vi "Stoerung Durchfluss FT-IR.vi"(10 "Durchfluss FT-IR":sgl) -> (0 "AbschMax":bool, 1 "AbschMin":bool, 2 "WarnMax":bool, 3 "WarnMin":bool, 5 "F.Br.":bool)   [LabVIEW 2020, in "Stoermeldungen.lvlib"]
uses:
  Stoermeldungen.lvlib
  Allgemein/FGV Analysator aktiv.ctl
  Aktion Anlagengrenzen pruefen.ctl
  Allgemein/FGV Zustaende Aktionen.ctl
  Seiten/Anlagengrenzwerte/Anlagen-Parameternamen.ctl
  Allgemein/Allgemein.lvlib
  Seiten/Anlagengrenzwerte/Anlagengrenzwerte.lvlib
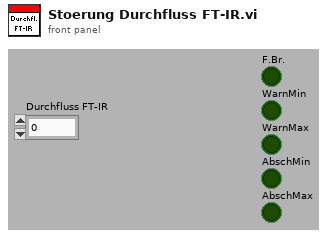
[diagram p1: front panel]
types:
  T1 = typedef "Allgemein.lvlib/FGV Analysator aktiv.ctl" = enum16{"lesen", "Analysator", "CG Aufschaltung", "KAL Zustand", "AutaKal GT?"}
  T2 = typedef "CalGas Aufschaltung.lvlib/Aufschaltung CalGas.ctl" = cluster{"Kalibriergas":T3, "Aufschaltpunkt":T4, "Analysator":T5}
  T3 = typedef "Auswahlfeld.ctl" = u16
  T4 = typedef "CalGas Aufschaltung.lvlib/Auswahl Aufschaltpunkt.ctl" = enum16{"über Filterblock", "Analysator direkt", "über PNS", "Entnahme", "Gasdivider"}
  T5 = typedef "CalGas Aufschaltung.lvlib/Auswahl Analysator.ctl" = enum16{"FT-IR", "FID", "PMA", "PMA/FID/FT-IR"}
  T6 = typedef "Status Analysatoren.lvlib/Status Analysatoren_Anzeige.ctl" = cluster{"FT-IR":bool, "FID":bool, "PMA":bool}
  T7 = typedef "Anlagengrenzwerte.lvlib/Anlagen-Parameternamen.ctl" = enum16{"Eingangsdruck FT-IR:", "Durchfluss FT-IR:", "Durchfluss CalGas", "Druck Ausgang", "Druck Kalter Block", "Heizleitung intern", "Heizleitung zu FT-IR", "Heizung Filter:", "Heizung Pumpe:", "HL Extern SP1", "HL Extern SP2", "FT-IR Messzelle", "Schaltschrank", "Gaskühler"}
  T8 = typedef "Allgemein.lvlib/FGV Zustaende Aktionen.ctl" = enum16{"lesen", "Zustand PC", "Zustand cRIO", "Bildnummer", "Samplepoint", "Sysloglevel"}
  T9 = typedef "Stoermeldungen.lvlib/Aktion Anlagengrenzen pruefen.ctl" = enum16{"Temp.", "HKL", "Druck", "SS Temp."}
  T10 = typedef "Funktionstasten.lvlib/Zustaende.ctl" = enum16{"Standby", "Pause", "Eco", "Messen", "Kalibrieren", "Spülen Filter", "Spülen Leitung", "Umgebungsluft", "0-Gas", "Cal-Gas", "CG zu PNS", "-------------", "Init 1", "Init 2", "Init 3", "Init 4", "Messen vorbereiten", "Messen durchführen", "Exit"}
  T11 = typedef "Auto Kalibrieren.lvlib/KalibrierZustaende.ctl" = cluster{"FTIR Zustand":u16, "PMA Zustand":u16, "FID CH4 Zustand":u16, "FID THC Zustand":u16, "FID THC CG":u16}
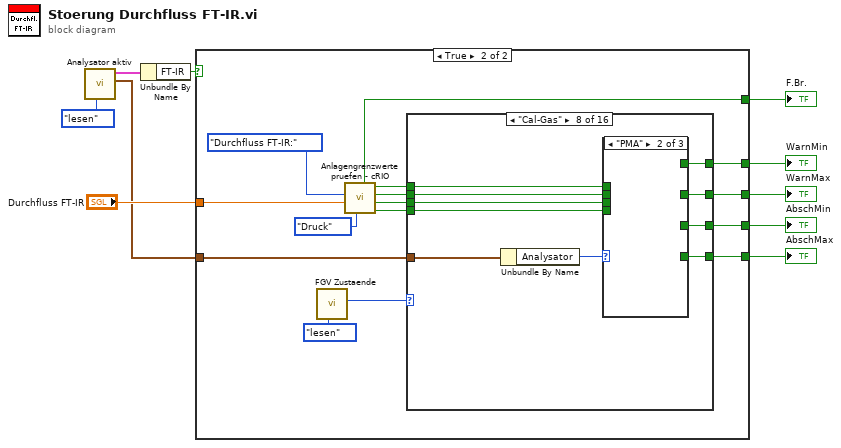
[diagram p0: block diagram]
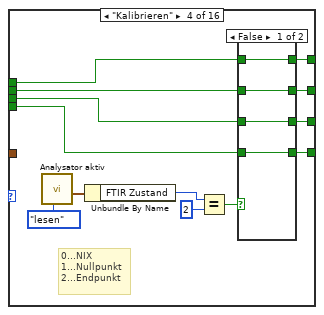
[diagram p6: hidden frame]
diagram:
  n1 = call "Analysator aktiv.vi"("Aktion"=FGV_Analysator_aktiv."lesen") -> ("Aufschaltung CalGas"=w2:T2, "Status Analysatoren"=w3:T6)  [unwired: 7 in, 2 out]
  n2 = Unbundle By Name(w3) -> ("FT-IR"=w8:bool)
  n3 = case shown="True" w8 {
    tunnel: "Durchfluss FT-IR" -> [_ w24]
    tunnel: [_ w23] -> w9
    tunnel: [_ w18] -> w7
    tunnel: [_ w17] -> w6
    tunnel: [_ w16] -> w5
    tunnel: [_ w15] -> w4
    tunnel: w2 -> [_ w12]
    frame False {
    }
    frame True {
      n4 = call "FGV Zustaende.vi"("Aktionen"=FGV_Zustaende_Aktionen."lesen") -> ("Zustand cRIO"=w13:T10)  [unwired: 6 in, 4 out]
      n5 = call "Anlagengrenzwerte pruefen - cRIO.vi"("Aktion"=Aktion_Anlagengrenzen_pruefen."Druck", "Wert"=w24, "Anlagen-Parametername"=Anlagen-Parameternamen."Durchfluss FT-IR:") -> ("AbschMax"=w19:bool, "AbschMin"=w20:bool, "WarnMax"=w21:bool, "WarnMin"=w22:bool, "F.Br."=w23:bool)  [unwired: 4 in]
      n6 = case shown="\"Cal-Gas\"" w13 {
        tunnel: w22 -> [_ _ w29 w37 _ _ w50 w59 _ _ _ _ _ _ _ _]
        tunnel: w21 -> [_ _ w28 w36 _ _ w49 w58 _ _ _ _ _ _ _ _]
        tunnel: w20 -> [_ _ w27 w35 _ _ w48 w57 _ _ _ _ _ _ _ _]
        tunnel: w19 -> [_ _ w26 w34 _ _ w47 w56 _ _ _ _ _ _ _ _]
        tunnel: [_ _ w29 w33 _ _ w50 w55 _ _ _ _ _ _ _ _] -> w18
        tunnel: [_ _ w28 w32 _ _ w49 w54 _ _ _ _ _ _ _ _] -> w17
        tunnel: [_ _ w27 w31 _ _ w48 w53 _ _ _ _ _ _ _ _] -> w16
        tunnel: [_ _ w26 w30 _ _ w47 w52 _ _ _ _ _ _ _ _] -> w15
        tunnel: w12 -> [_ _ _ _ _ _ _ w51 _ _ _ _ _ _ _ _]
        frame "Standby", Default {
        }
        frame "Pause" {
        }
        frame "Messen" {
        }
        frame "Kalibrieren" {
          # "0...NIX\n1...Nullpunkt\n2...Endpunkt"
          n7 = call "Analysator aktiv.vi"("Aktion"=FGV_Analysator_aktiv."lesen") -> ("Kalibrieren"=w40:T11)  [unwired: 7 in, 3 out]
          n8 = Unbundle By Name(w40) -> ("FTIR Zustand"=w41:u16)
          n9 = Equal?(x=w41, y=u16 2) -> (x = y?=w38:bool)
          n10 = case shown="False" w38 {
            tunnel: w37 -> [w46 _]
            tunnel: w36 -> [w45 _]
            tunnel: w35 -> [w44 _]
            tunnel: w34 -> [w43 _]
            tunnel: [w46 _] -> w33
            tunnel: [w45 _] -> w32
            tunnel: [w44 _] -> w31
            tunnel: [w43 _] -> w30
            frame False {
            }
            frame True {
            }
          }
        }
        frame "Spülen Filter" {
        }
        frame "Spülen Leitung" {
        }
        frame "0-Gas" {
        }
        frame "Cal-Gas" {
          n11 = Unbundle By Name(w51) -> ("Analysator"=w60:T5)
          n12 = case shown="\"PMA\"" w60 {
            tunnel: w59 -> [w64 _ _]
            tunnel: w58 -> [w63 _ _]
            tunnel: w57 -> [w62 _ _]
            tunnel: w56 -> [w61 _ _]
            tunnel: [w64 _ _] -> w55
            tunnel: [w63 _ _] -> w54
            tunnel: [w62 _ _] -> w53
            tunnel: [w61 _ _] -> w52
            frame "FT-IR", Default {
            }
            frame "PMA" {
            }
            frame "FID" {
            }
          }
        }
        frame "-------------" {
        }
        frame "Init 1" {
        }
        frame "Init 2" {
        }
        frame "Init 3" {
        }
        frame "Init 4" {
        }
        frame "Messen vorbereiten" {
        }
        frame "Messen durchführen" {
        }
        frame "Exit" {
        }
      }
    }
  }
  "F.Br." <- w9
  "WarnMin" <- w7
  "WarnMax" <- w6
  "AbschMin" <- w5
  "AbschMax" <- w4
